vi "Is LVJSON.vi"(1 "Variant":variant) -> (0 "Is LVJSON?":bool)   [LabVIEW 2019, in "labview_json.lvlib"]
uses:
  labview_json.lvlib
  <vilib>/Utility/Data Type/Type Definitions/Data Type.ctl
  <vilib>/Utility/Data Type/NI_Data Type.lvlib
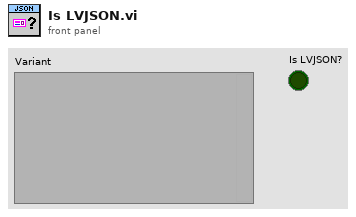
[diagram p1: front panel]
types:
  T1 = typedef "NI_Data Type.lvlib/Data Type.ctl" = enum8{"Invalid Type", "Void", "I8", "I16", "I32", "I64", "U8", "U16", "U32", "U64", "Single Float", "Double Float", "Extended Float", "Single Complex", "Double Complex", "Extended Complex", "Enum U8", "Enum U16", "Enum U32", "Enum U64", "Single Float With Unit", "Double Float With Unit", "Extended Float With Unit", "Single Complex with Unit", "Double Complex with Unit", "Extended Complex with Unit", "Boolean", "String", "Path", "Picture", "Tag", "Array", "Cluster", "Variant", "LV Variant", "Waveform", "Timestamp", "Digital Waveform", "Digital Data", "ExpressData", "Refnum", "External Data", "VI", "Poly VI", "LabVIEW Class Instance", "Fixed Point", "Set Collection", "Map Collection"}
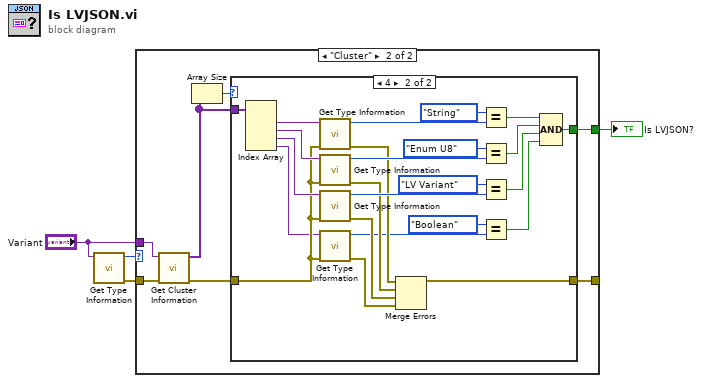
[diagram p0: block diagram]
diagram:
  n1 = call <vilib>:"Get Type Information.vi"("variant"="Variant") -> ("error out"=w4:errorcluster, "type"=w3:T1)  [unwired: 6 in, 3 out]
  n2 = case shown="\"Cluster\"" w3 {
    tunnel: "Variant" -> [_ w12]
    tunnel: [_ w9] -> w1
    tunnel: w4 -> [w5 w8]
    tunnel: [w5 w6] -> _
    frame Default {
    }
    frame "Cluster" {
      n3 = call <vilib>:"Get Cluster Information.vi"("error in (no error)"=w8, "variant"=w12) -> ("error out"=w7:errorcluster, "cluster elements"=w10:variant[])  [unwired: 8 in]
      n4 = Array Size(array=w10) -> (size(s)=w11:i32)
      n5 = case shown="4" w11 {
        tunnel: w10 -> [_ w37]
        tunnel: [_ w33] -> w9
        tunnel: w7 -> [w13 w17]
        tunnel: [w13 w32] -> w6
        frame Default {
        }
        frame 4 {
          n6 = Index Array(array=w37) -> (element #1=w24:variant, element #2=w26:variant, element #3=w27:variant, element #4=w16:variant)  [unwired: 4 in]
          n7 = call <vilib>:"Get Type Information.vi"("error in (no error)"=w17, "variant"=w24) -> ("error out"=w25:errorcluster, "type"=w23:T1)  [unwired: 5 in, 3 out]
          n8 = call <vilib>:"Get Type Information.vi"("error in (no error)"=w17, "variant"=w26) -> ("error out"=w29:errorcluster, "type"=w28:T1)  [unwired: 5 in, 3 out]
          n9 = call <vilib>:"Get Type Information.vi"("error in (no error)"=w17, "variant"=w27) -> ("error out"=w31:errorcluster, "type"=w30:T1)  [unwired: 5 in, 3 out]
          n10 = call <vilib>:"Get Type Information.vi"("error in (no error)"=w17, "variant"=w16) -> ("error out"=w14:errorcluster, "type"=w18:T1)  [unwired: 5 in, 3 out]
          n11 = Merge Errors(w25, w29, w31, w14) -> (w32:errorcluster)
          n12 = Equal?(x=Data_Type."String" ("Type"), y=w23) -> (x = y?=w36:bool)
          n13 = Equal?(x=Data_Type."Enum U8" ("Type"), y=w28) -> (x = y?=w35:bool)
          n14 = Equal?(x=Data_Type."LV Variant" ("Type"), y=w30) -> (x = y?=w34:bool)
          n15 = Equal?(x=Data_Type."Boolean" ("Type"), y=w18) -> (x = y?=w15:bool)
          n16 = Compound Arithmetic op=AND(w36, w35, w34, w15) -> (w33:bool)
        }
      }
    }
  }
  "Is LVJSON?" <- w1
